vi "PV ActiveLine - KeyboardTest.vi"(8 "Fehler (Eingang)":errorcluster, 11 "Referenz in":refnum<visa-resource-name>) -> (0 "Cluster (Ausgang)":errorcluster, 1 "Key 3":i32(ring) items=["Not pushed", "pushed"], 2 "Key 2":i32(ring) items=["Not pushed", "pushed"], 3 "Referenz out":refnum<visa-resource-name>, 4 "Key 4":i32(ring) items=["Not pushed", "pushed"], 5 "Key 1":i32(ring) items=["Not pushed", "pushed"])   [LabVIEW 2013, in "PV ActiveLine.lvlib"]
doc: "TKB - Operator Key Test\n\nReceive: abcd\n\nKey 1,\na =\n0 –> Not pushed\n1 –> Pushed\n\nKey 2,\nb =\n0 –> Not pushed\n1 –> Pushed\n\nKey 3,\nc =\n0 –> Not pushed\n1 –> Pushed\n\nKey 4,\nd =\n0 –> Not pushed\n1 –> Pushed"
uses:
  <instrlib>/PV ActiveLine/PV ActiveLine.lvlib
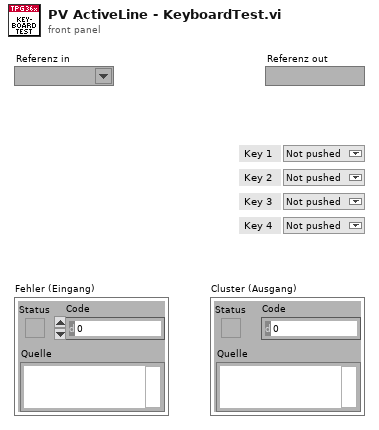
[diagram p1: front panel]
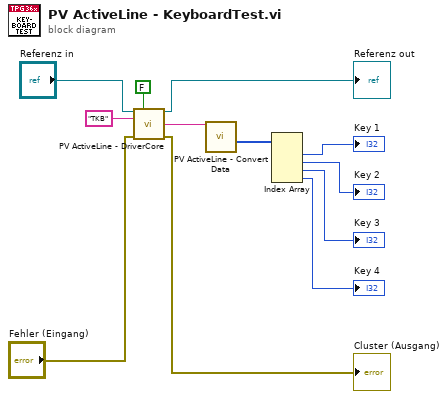
[diagram p0: block diagram]
diagram:
  n1 = call <instrlib>:"PV ActiveLine - DriverCore.vi"("Referenz in"="Referenz in", "Write/Read"=FALSE ("W/R"), "Command"="TKB", "Fehler (Eingang)"="Fehler (Eingang)") -> ("Referenz out"=→"Referenz out":refnum<visa-resource-name>, "String Out"=w6:string, "Cluster (Ausgang)"=→"Cluster (Ausgang)":errorcluster)  [unwired: 9 in]
  n2 = call <instrlib>:"PV ActiveLine - Convert Data.vi"("String in"=w6) -> ("Integer Out"=w5:i32[])  [unwired: 7 in, 3 out]
  n3 = Index Array(array=w5) -> (element #1=→"Key 1":i32, element #2=→"Key 2":i32, element #3=→"Key 3":i32, element #4=→"Key 4":i32)  [unwired: 4 in]
